vi "Run Test Case.vi"(8 "error in (no error)":errorcluster, 11 "VI Refnum":refnum<vi>) -> (0 "error out":errorcluster, 3 "VI Refnum out":refnum<vi>)   [LabVIEW 2017, in "LVUnit Test Executor.lvclass"]
uses:
  LVUnit Test Executor.lvclass
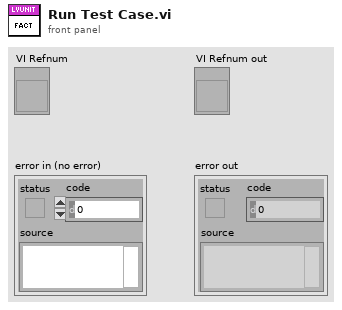
[diagram p1: front panel]
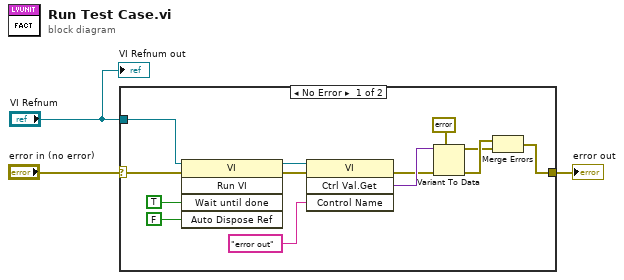
[diagram p0: block diagram]
diagram:
  n1 = case shown="No Error" "error in (no error)" {
    selector: "error in (no error)" -> [w5 w17]
    tunnel: [w6 w17] -> w2
    tunnel: "VI Refnum" -> [w4 _]
    frame No Error {
      n2 = invoke class="VI" method="Run VI"(reference=w4, error in=w5, "Wait until done"=TRUE ("Wait Until Done"), "Auto Dispose Ref"=FALSE ("Auto Dispose Reference")) -> (reference out=w13:refnum<vi>, error out=w12:errorcluster)  [unwired: 1 in, 3 out]
      n3 = invoke class="VI" method="Ctrl Val.Get"(reference=w13, error in=w12, "Control Name"="error out") -> (error out=w7:errorcluster, "Get Control Value Variant"=w10:variant)  [unwired: 1 in, 2 out]
      n4 = Variant To Data(error in=w7, type=errorcluster {"status"=FALSE, "code"=0, "source"=""}, Variant=w10) -> (data=w8:errorcluster, error out=w11:errorcluster)
      n5 = Merge Errors(w11, w8) -> (w6:errorcluster)
    }
    frame Error {
    }
  }
  "error out" <- w2
  "VI Refnum out" <- "VI Refnum"
